vi "TimeFlow_for_泰克.vi"() -> ()   [LabVIEW 2017]
uses:
  <vilib>/vision/Image Controls.llb/IMAQ Image.ctl
  <vilib>/userdefined/High Color/IMAQdx.ctl
  <vilib>/vision/driver/IMAQdx.llb/IMAQdx Camera Control Mode.ctl
  <vilib>/Utility/file.llb/Write Delimited Spreadsheet (I64).vi
  <vilib>/vision/driver/NI_Vision_Acquisition_Software.lvlib
  <vilib>/vision/NI_Vision_Development_Module.lvlib
panel:
  in  "EOT reset":bool=TRUE
  out "DO 4":bool
  out "DO 2":bool
  out "DO 0":bool
  out "None":dbl
  out "Total":dbl
  out "No sample":dbl
  out "NG":dbl
  out "PASS":dbl
  in  "SOT single trigger":bool
  in  "SOT inverse":bool
  out "code":u32
  in  "Camera port":T1="cam1"
  in  "No sample":bool
  in  "NG":bool
  in  "EOT inverse":bool
  out "EOT":bool
  in  "CCD 啟動":bool
  out "EOT切換2":bool
  out "結果":bool
  out "檢查":bool
  out "EOT切換1":bool
  out "SOT等待":bool
  out "SOT":bool
  in  "EOT Run End":bool=TRUE
  in  "EOT Run State":bool
  in  "EOT Start State":bool=TRUE
  in  "physical channels":string="PCI-1730,BID#0"
  in  "儲存DATA":bool
  in  "儲存IMAGE":bool
  in  "清除":bool
  out "Show":u32[](graph)
  out "Time":T2
  in  "EOT DELAY":u32=20
  in  "Pass":bool=TRUE
  in  "虛擬檢測時間":u32=5
  in  "等待拍照":u32=13
  in  "SOT DELAY":u32
  in  "與機台連線":bool=TRUE
  out "New Image":T3
  in  "連續取像":bool=TRUE
  in  "Angle (degrees)":sgl format="%.2f"
  out "Image":T3(plugin-control)
  in  "error in":errorcluster
  in  "stop":bool
  out "IO status":bool
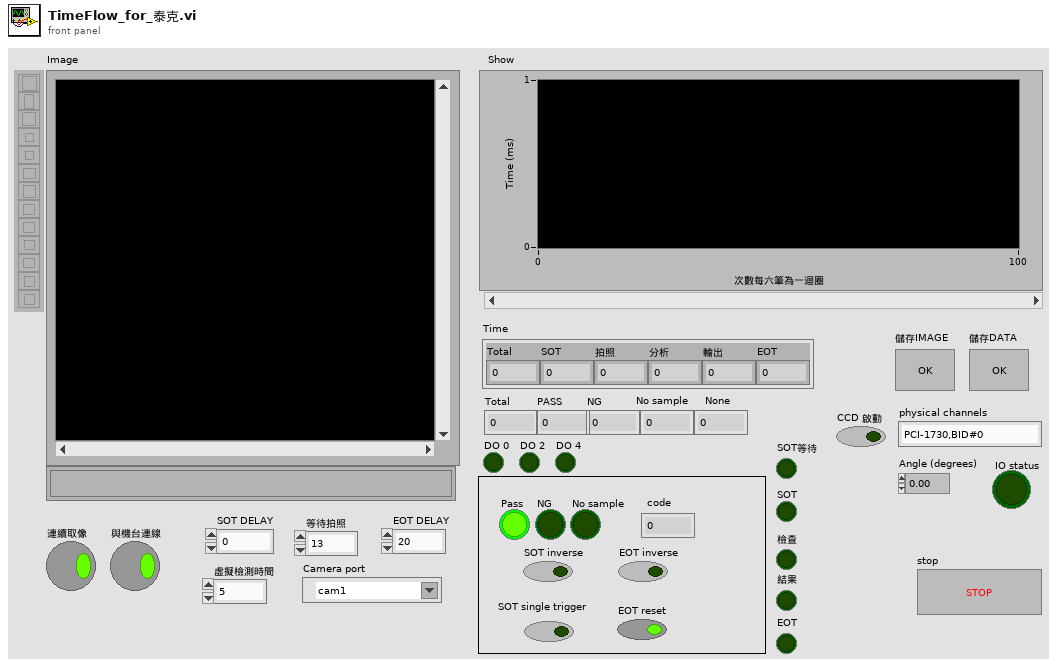
[diagram p1: front panel]
types:
  T1 = typedef "IMAQdx.ctl" = refnum<k21>
  T2 = cluster{"Total":dbl, "SOT":dbl, "拍照":dbl, "分析":dbl, "輸出":dbl, "EOT":dbl}
  T3 = typedef "IMAQ Image.ctl" = refnum<image>
  T4 = typedef "NI_Vision_Acquisition_Software.lvlib/IMAQdx Camera Control Mode.ctl" = enum32{"Controller", "Listener"}
  T5 = typedef "Image Type" = u32
  T6 = cluster{"task DI 0~7":i32, "portBit":i32, "Boolean out":bool}
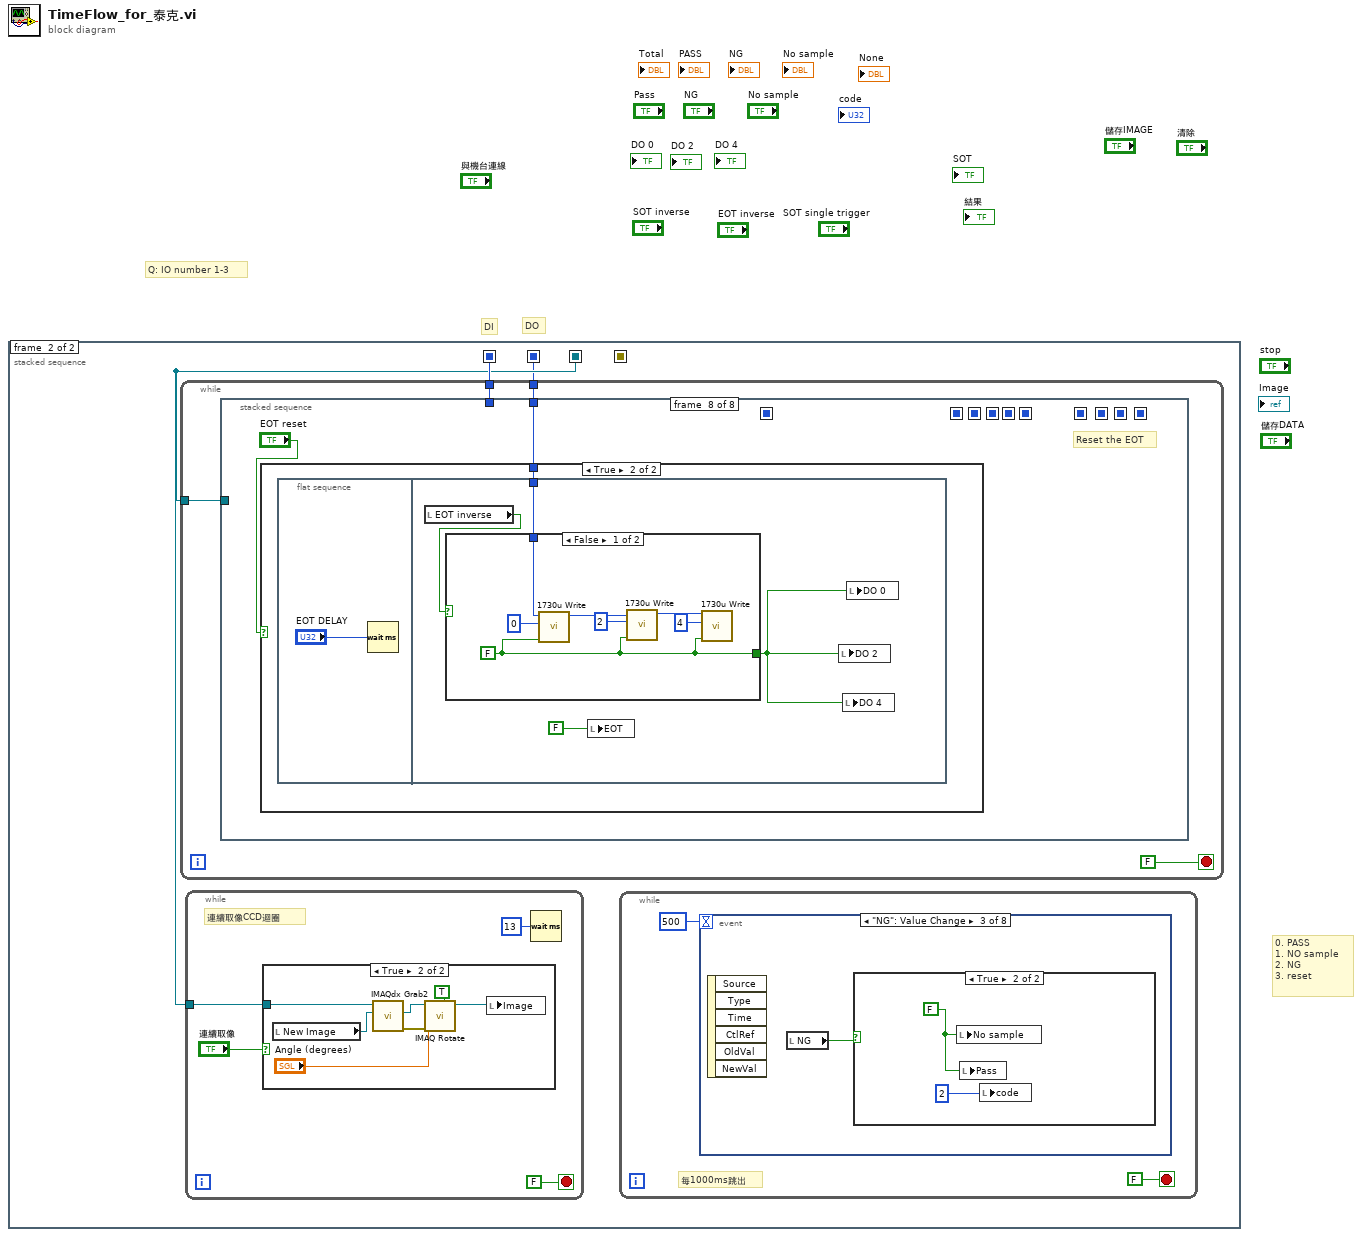
[diagram p0: block diagram]
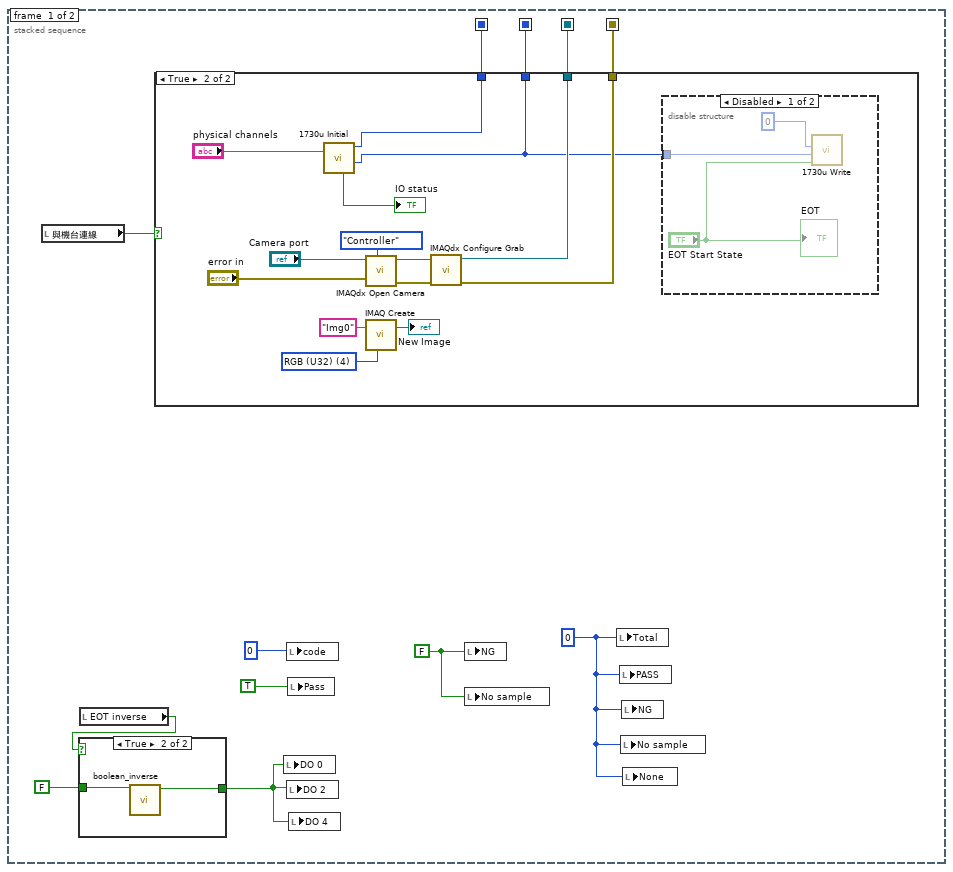
[diagram p2: hidden frame]
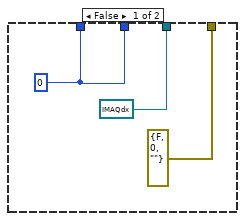
[diagram p4: hidden frame]
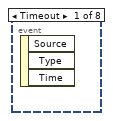
[diagram p6: hidden frame]
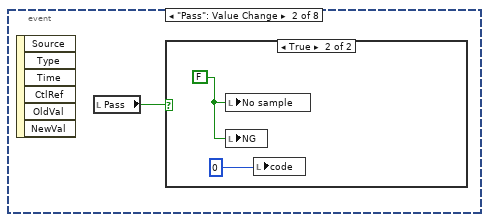
[diagram p7: hidden frame]
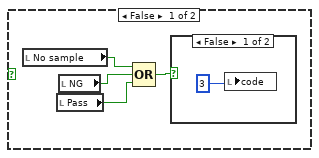
[diagram p8: hidden frame]
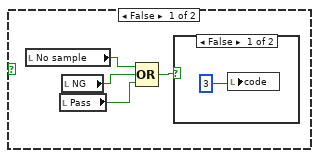
[diagram p10: hidden frame]
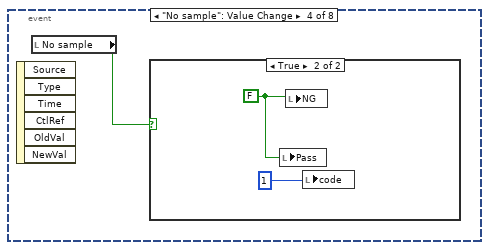
[diagram p12: hidden frame]
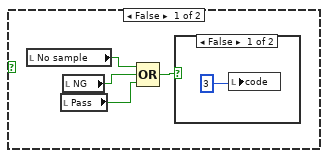
[diagram p13: hidden frame]
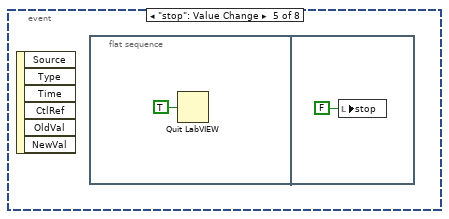
[diagram p15: hidden frame]
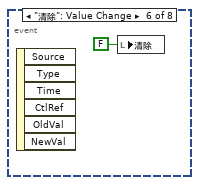
[diagram p16: hidden frame]
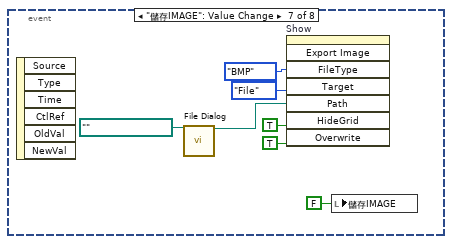
[diagram p17: hidden frame]
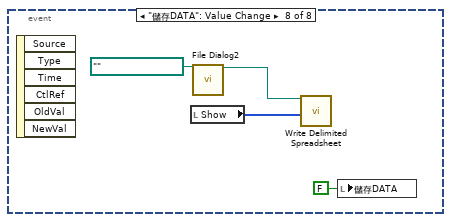
[diagram p18: hidden frame]
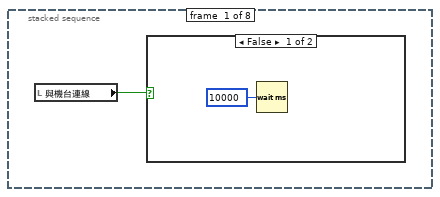
[diagram p20: hidden frame]
diagram:
  # "0. PASS\n1. NO sample\n2. NG\n3. reset"
  # "Q: IO number 1-3"
  # "DO"
  # "DI"
  n1 = stacked-sequence {
    seq-local: [w12 _] -> [_ w38]
    seq-local: [w9 _] -> [_ w36]
    seq-local: [w11 _] -> [_ _]
    seq-local: [w10 _] -> [_ w37]
    frame #0 {
      w5 = 0
      w8 = FALSE
      n2 = local read "與機台連線"() -> (w7:bool)
      n3 = local read "EOT inverse"() -> (w2:bool)
      n4 = case shown="True" w2 {
        tunnel: FALSE -> [w13 w15]
        tunnel: [w13 w14] -> w1
        frame False {
        }
        frame True {
          n5 = call "boolean_inverse.vi"("Boolean in"=w15) -> ("Boolean out"=w14:bool)  [unwired: 10 in]
        }
      }
      n6 = case shown="True" w7 {
        tunnel: [w18 w32] -> w12
        tunnel: [errorcluster {"status"=FALSE, "code"=0, "source"=""} ("error out") w31] -> w11
        tunnel: [T1 refnum ("Session Out") w30] -> w10
        tunnel: [w18 w29] -> w9
        frame False {
          w18 = 0
        }
        frame True {
          w21 = T5 4 items=["Grayscale (U8)", "Grayscale (I16)", "Grayscale (SGL)", "Complex (CSG)", "RGB (U32)", "HSL (U32)", "RGB (U64)", "Grayscale (U16)"] ("Image Type")
          n7 = call <userlib>:"1730u Initial.vi"("physical channels"="physical channels") -> ("task DO 0~7"=w29:i32, "task DI 0~7"=w32:i32, "status"=→"IO status":bool)  [unwired: 6 in, 2 out]
          n8 = call <vilib>:"IMAQdx Open Camera.vi"("Camera Control Mode"=IMAQdx_Camera_Control_Mode."Controller", "error in"="error in", "Session In"="Camera port") -> ("error out"=w25:errorcluster, "Session Out"=w26:T1)  [unwired: 7 in]
          n9 = call "IMAQ Create"("Image Name"="Img0", "Image Type"=w21) -> ("New Image"=→"New Image":T3)  [unwired: 3 in, 1 out]
          n10 = call <vilib>:"IMAQdx Configure Grab.vi"("error in"=w25, "Session In"=w26) -> ("error out"=w31:errorcluster, "Session Out"=w30:T1)  [unwired: 8 in]
          n11 = disable-structure shown="Disabled" {
            disable-tunnel: w29 -> [w34 _]
            frame Disabled {
              n12 = call <userlib>:"1730u Write.vi"("data"="EOT Start State", "portBit"=0, "DO task in"=w34) -> ()  [unwired: 8 in, 1 out]
              "EOT" <- "EOT Start State"
            }
            frame Enabled {
            }
          }
        }
      }
      n13 = local write "DO 0"(w1) -> ()
      n14 = local write "code"(0) -> ()
      n15 = local write "DO 2"(w1) -> ()
      n16 = local write "Pass"(TRUE) -> ()
      n17 = local write "DO 4"(w1) -> ()
      n18 = local write "NG"(w8) -> ()
      n19 = local write "No sample"(w8) -> ()
      n20 = local write "Total"(w5) -> ()
      n21 = local write "PASS"(w5) -> ()
      n22 = local write "No sample"(w5) -> ()
      n23 = local write "NG"(w5) -> ()
      n24 = local write "None"(w5) -> ()
    }
    frame #1 {
      n25 = while {
        tunnel: w38 -> [w92]
        tunnel: w37 -> [w91]
        tunnel: w36 -> [w90]
        stop <- FALSE stop-if-true
        n26 = stacked-sequence {
          seq-local: [_ w99 _ _ _ _ _ _] -> [_ _ w138 _ _ _ w269 _]
          seq-local: [_ _ w137 _ _ _ _ _] -> [_ _ _ _ _ _ w265 _]
          seq-local: [_ _ w136 _ _ _ _ _] -> [_ _ _ w145 _ _ _ _]
          seq-local: [_ _ _ w143 _ _ _ _] -> [_ _ _ _ _ _ w264 _]
          seq-local: [_ _ _ w141 _ _ _ _] -> [_ _ _ _ w189 _ _ _]
          seq-local: [_ _ _ _ w178 _ _ _] -> [_ _ _ _ _ w226 _ _]
          seq-local: [_ _ _ _ w188 _ _ _] -> [_ _ _ _ _ _ w263 _]
          seq-local: [_ _ _ _ w187 _ _ _] -> [_ _ _ _ _ w224 _ _]
          seq-local: [_ _ _ _ _ w223 _ _] -> [_ _ _ _ _ _ w262 _]
          seq-local: [_ _ _ _ _ w222 _ _] -> [_ _ _ _ _ _ w267 _]
          tunnel: w92 -> [_ w100 _ _ _ w219 _ _]
          tunnel: w91 -> [_ _ _ w148 _ _ _ _]
          tunnel: w90 -> [_ w98 _ _ w176 _ _ w271]
          frame #0 {
            n27 = local read "與機台連線"() -> (w94:bool)
            n28 = case shown="False" w94 {
              frame False {
                n29 = Wait (ms)(milliseconds to wait=u32 10000) -> ()  [unwired: 1 out]
              }
              frame True {
              }
            }
          }
          frame #1 {
            # "Double reset the EOT"
            # "IO"
            n30 = flat-sequence {
              tunnel: w100 -> [w103]
              tunnel: [w102] -> w99
              frame #0 {
                n31 = Wait (ms)(milliseconds to wait="SOT DELAY") -> ()  [unwired: 1 out]
              }
              frame #1 {
                n32 = while {
                  tunnel: w103 -> [w115]
                  tunnel: [w113] -> w102
                  stop <- w114 stop-if-true
                  n33 = call <userlib>:"1730u Read.vi"("portBit"=0, "DI task in"=w115) -> ("data"=w107:bool)  [unwired: 8 in, 1 out]
                  n34 = local write "EOT切換2"(FALSE ("EOT切換2")) -> ()
                  n35 = local read "SOT single trigger"() -> (w106:bool)
                  n36 = local read "SOT inverse"() -> (w108:bool)
                  n37 = case shown="True" w108 {
                    tunnel: w107 -> [w116 w118]
                    tunnel: [w116 w117] -> w105
                    frame False {
                    }
                    frame True {
                      n38 = call "boolean_inverse.vi"("Boolean in"=w118) -> ("Boolean out"=w117:bool)  [unwired: 10 in]
                    }
                  }
                  n39 = local read "與機台連線"() -> (w110:bool)
                  n40 = Or(x=w106, y=w105) -> (x .or. y?=w104:bool)
                  n41 = And(x=w104, y=w110) -> (x .and. y?=w114:bool)
                  n42 = local write "SOT"(w104) -> ()
                  n43 = case shown="True" w114 {
                    tunnel: [u32 0 ("millisecond timer value") w120] -> w113
                    frame False {
                    }
                    frame True {
                      n44 = Tick Count (ms)() -> (millisecond timer value=w120:u32)
                    }
                  }
                  "SOT等待" <- TRUE ("SOT等待")
                }
              }
            }
            n45 = local read "EOT inverse"() -> (w97:bool)
            n46 = case shown="False" w97 {
              tunnel: w98 -> [w122 w131]
              tunnel: [w121 w128] -> w96
              frame False {
                w121 = FALSE ("data")
                n47 = call <userlib>:"1730u Write.vi"("data"=w121, "portBit"=0, "DO task in"=w122) -> ("DO task out"=w127:i32)  [unwired: 8 in]
                n48 = call <userlib>:"1730u Write.vi"("data"=w121, "portBit"=2, "DO task in"=w127) -> ("DO task out"=w126:i32)  [unwired: 8 in]
                n49 = call <userlib>:"1730u Write.vi"("data"=w121, "portBit"=4, "DO task in"=w126) -> ()  [unwired: 8 in, 1 out]
              }
              frame True {
                w128 = TRUE ("data")
                n50 = call <userlib>:"1730u Write.vi"("data"=w128, "portBit"=0, "DO task in"=w131) -> ("DO task out"=w133:i32)  [unwired: 8 in]
                n51 = call <userlib>:"1730u Write.vi"("data"=w128, "portBit"=2, "DO task in"=w133) -> ("DO task out"=w129:i32)  [unwired: 8 in]
                n52 = call <userlib>:"1730u Write.vi"("data"=w128, "portBit"=4, "DO task in"=w129) -> ()  [unwired: 8 in, 1 out]
              }
            }
            n53 = local write "DO 2"(w96) -> ()
            n54 = local write "DO 0"(w96) -> ()
            n55 = local write "DO 4"(w96) -> ()
          }
          frame #2 {
            w135 = FALSE ("SOT等待")
            n56 = Wait (ms)(milliseconds to wait="等待拍照") -> ()  [unwired: 1 out]
            n57 = local write "SOT等待"(w135) -> ()
            n58 = local write "SOT single trigger"(w135) -> ()
            n59 = Tick Count (ms)() -> (millisecond timer value=w136:u32)
            n60 = Subtract(x=w136, y=w138) -> (x-y=w137:u32)
          }
          frame #3 {
            n61 = flat-sequence {
              tunnel: w148 -> [w156]
              tunnel: [w155] -> w147
              tunnel: [w154] -> w146
              tunnel: w145 -> [w153]
              tunnel: [w152] -> w144
              tunnel: [w151] -> w142
              tunnel: [w168] -> w143
              tunnel: [w166] -> w141
              tunnel: w142 -> [w166]
              tunnel: w144 -> [w168]
              tunnel: w146 -> [_]
              tunnel: w147 -> [w169]
              frame #0 {
                # "CCD"
                n62 = local read "New Image"() -> (w149:T3)
                n63 = case shown="True" "CCD 啟動" {
                  tunnel: w156 -> [_ w165]
                  tunnel: [w157 w161] -> w155
                  tunnel: [errorcluster {"status"=FALSE, "code"=0, "source"=""} ("error out") w160] -> w154
                  tunnel: w149 -> [w157 w159]
                  frame False {
                  }
                  frame True {
                    n64 = local read "Angle (degrees)"() -> (w162:sgl)
                    n65 = call <vilib>:"IMAQdx Grab2.vi"("Image In"=w159, "Session In"=w165) -> ("error out"=w163:errorcluster, "Image Out"=w164:T3)  [unwired: 6 in, 2 out]
                    n66 = call "IMAQ Rotate"("error in (no error)"=w163, "Angle (degrees)"=w162, "Image Src"=w164) -> ("error out"=w160:errorcluster, "Image Dst Out"=w161:T3)  [unwired: 7 in]
                  }
                }
                n67 = Tick Count (ms)() -> (millisecond timer value=w151:u32)
                n68 = Subtract(x=w151, y=w153) -> (x-y=w152:u32)
              }
              frame #1 {
                # "Set the runtime for algorithm"
                n69 = local write "Image"(w169) -> ()
                n70 = Wait (ms)(milliseconds to wait="虛擬檢測時間") -> ()  [unwired: 1 out]
              }
            }
            "檢查" <- TRUE ("檢查")
          }
          frame #4 {
            n71 = local read "code"() -> (w185:u32)
            n72 = local write "檢查"(FALSE ("檢查")) -> ()
            n73 = local write "結果"(TRUE ("結果")) -> ()
            n74 = case shown="0, Default" w185 {
              tunnel: [TRUE TRUE TRUE FALSE] -> w184
              tunnel: [FALSE TRUE TRUE FALSE] -> w183
              tunnel: [FALSE TRUE FALSE FALSE] -> w182
              frame 0, Default {
                n75 = local read "PASS"() -> (w200:dbl)
                n76 = Increment(x=w200) -> (x+1=w199:dbl)
                n77 = local write "PASS"(w199) -> ()
              }
              frame 1 {
                n78 = local read "No sample"() -> (w204:dbl)
                n79 = Increment(x=w204) -> (x+1=w205:dbl)
                n80 = local write "No sample"(w205) -> ()
              }
              frame 2 {
                n81 = local read "NG"() -> (w210:dbl)
                n82 = Increment(x=w210) -> (x+1=w209:dbl)
                n83 = local write "NG"(w209) -> ()
              }
              frame 3 {
                n84 = local read "None"() -> (w214:dbl)
                n85 = Increment(x=w214) -> (x+1=w215:dbl)
                n86 = local write "None"(w215) -> ()
              }
            }
            n87 = local read "EOT inverse"() -> (w177:bool)
            n88 = case shown="True" w177 {
              tunnel: w184 -> [w192 w198]
              tunnel: [w192 w197] -> w170
              tunnel: w183 -> [w191 w196]
              tunnel: [w191 w195] -> w171
              tunnel: w182 -> [w190 w194]
              tunnel: [w190 w193] -> w172
              frame False {
              }
              frame True {
                n89 = call "boolean_inverse.vi"("Boolean in"=w198) -> ("Boolean out"=w197:bool)  [unwired: 10 in]
                n90 = call "boolean_inverse.vi"("Boolean in"=w196) -> ("Boolean out"=w195:bool)  [unwired: 10 in]
                n91 = call "boolean_inverse.vi"("Boolean in"=w194) -> ("Boolean out"=w193:bool)  [unwired: 10 in]
              }
            }
            n92 = call <userlib>:"1730u Write.vi"("data"=w172, "portBit"=4, "DO task in"=w176) -> ()  [unwired: 8 in, 1 out]
            n93 = call <userlib>:"1730u Write.vi"("data"=w171, "portBit"=2, "DO task in"=w176) -> ()  [unwired: 8 in, 1 out]
            n94 = call <userlib>:"1730u Write.vi"("data"=w170, "portBit"=0, "DO task in"=w176) -> ("DO task out"=w178:i32)  [unwired: 8 in]
            n95 = local write "DO 2"(w171) -> ()
            n96 = local write "DO 4"(w172) -> ()
            n97 = local write "DO 0"(w170) -> ()
            n98 = Tick Count (ms)() -> (millisecond timer value=w187:u32)
            n99 = Subtract(x=w187, y=w189) -> (x-y=w188:u32)
            n100 = local read "Total"() -> (w173:dbl)
            n101 = Increment(x=w173) -> (x+1=w174:dbl)
            n102 = local write "Total"(w174) -> ()
          }
          frame #5 {
            n103 = flat-sequence {
              tunnel: w219 -> [w229]
              tunnel: w226 -> [w228]
              tunnel: [w227] -> w221
              tunnel: [w229] -> w220
              tunnel: [w235] -> w225
              tunnel: w221 -> [w236]
              tunnel: w220 -> [w235]
              tunnel: w225 -> [w248]
              frame #0 {
                n104 = disable-structure shown="Disabled" {
                  disable-tunnel: w228 -> [w232 _]
                  disable-tunnel: [w231 _] -> w227
                  frame Disabled {
                    n105 = local write "EOT"("EOT Run State") -> ()
                    n106 = call <userlib>:"1730u Write.vi"("data"="EOT Run State", "portBit"=0, "DO task in"=w232) -> ("DO task out"=w231:i32)  [unwired: 8 in]
                    "EOT切換1" <- TRUE ("EOT切換1")
                  }
                  frame Enabled {
                  }
                }
              }
              frame #1 {
                n107 = disable-structure shown="Disabled" {
                  disable-tunnel: w236 -> [w240 _]
                  frame Disabled {
                    n108 = local write "結果"(FALSE ("結果")) -> ()
                    n109 = local write "EOT"("EOT Run End") -> ()
                    n110 = call <userlib>:"1730u Write.vi"("data"="EOT Run End", "portBit"=0, "DO task in"=w240) -> ()  [unwired: 8 in, 1 out]
                    "EOT切換2" <- TRUE ("EOT切換2")
                  }
                  frame Enabled {
                  }
                }
              }
              frame #2 {
                n111 = local read "SOT inverse"() -> (w244:bool)
                n112 = case shown="True" w244 {
                  tunnel: FALSE -> [w254 w256]
                  tunnel: [w254 w255] -> w243
                  frame False {
                  }
                  frame True {
                    n113 = call "boolean_inverse.vi"("Boolean in"=w256) -> ("Boolean out"=w255:bool)  [unwired: 10 in]
                  }
                }
                n114 = Bundle("task DI 0~7"=w248, "portBit"=0, "Boolean out"=w243) -> (w247:T6)  [unwired: 1 in]
                n115 = local write "EOT"(TRUE ("EOT切換1")) -> ()
                n116 = call <userlib>:"Check DI State 1730u.vi"("Time Out"=u32 3000 ("DI Time Out"), "Scan time"=u32 2 ("DI Scan time"), "Mode"=enum16{"Check One DI", "Check Two DI"}."Check One DI", "1 DI Mode"=w247) -> ("Finish?"=w253:bool)  [unwired: 7 in]
                n117 = local write "結果"(FALSE) -> ()
                n118 = case shown="True" w253 {
                  frame False {
                    n119 = One Button Dialog(message="SOT持續超過3秒\n沒有關閉") -> ()  [unwired: 1 in, 1 out]
                  }
                  frame True {
                    n120 = local write "SOT"(FALSE ("檢查")) -> ()
                  }
                }
              }
            }
            n121 = Tick Count (ms)() -> (millisecond timer value=w222:u32)
            n122 = Subtract(x=w222, y=w224) -> (x-y=w223:u32)
          }
          frame #6 {
            n123 = Tick Count (ms)() -> (millisecond timer value=w268:u32)
            n124 = Subtract(x=w268, y=w269) -> (x-y=w266:u32)
            n125 = Subtract(x=w268, y=w267) -> (x-y=w261:u32)
            n126 = Bundle(w266, w265, w264, w263, w262, w261) -> (w260:cluster{u32, u32, u32, u32, u32, u32})  [unwired: 1 in]
            "Time" <- w260
            n127 = Cluster To Array(cluster=w260) -> (array=→"Show":u32[])
          }
          frame #7 {
            # "Reset the EOT"
            n128 = case shown="True" "EOT reset" {
              tunnel: w271 -> [_ w272]
              frame False {
              }
              frame True {
                n129 = flat-sequence {
                  tunnel: w272 -> [w277]
                  frame #0 {
                    n130 = Wait (ms)(milliseconds to wait="EOT DELAY") -> ()  [unwired: 1 out]
                  }
                  frame #1 {
                    n131 = local read "EOT inverse"() -> (w276:bool)
                    n132 = case shown="False" w276 {
                      tunnel: w277 -> [w279 w286]
                      tunnel: [w278 w285] -> w274
                      frame False {
                        w278 = FALSE ("data")
                        n133 = call <userlib>:"1730u Write.vi"("data"=w278, "portBit"=0, "DO task in"=w279) -> ("DO task out"=w284:i32)  [unwired: 8 in]
                        n134 = call <userlib>:"1730u Write.vi"("data"=w278, "portBit"=2, "DO task in"=w284) -> ("DO task out"=w283:i32)  [unwired: 8 in]
                        n135 = call <userlib>:"1730u Write.vi"("data"=w278, "portBit"=4, "DO task in"=w283) -> ()  [unwired: 8 in, 1 out]
                      }
                      frame True {
                        w285 = TRUE ("data")
                        n136 = call <userlib>:"1730u Write.vi"("data"=w285, "portBit"=0, "DO task in"=w286) -> ("DO task out"=w291:i32)  [unwired: 8 in]
                        n137 = call <userlib>:"1730u Write.vi"("data"=w285, "portBit"=2, "DO task in"=w291) -> ("DO task out"=w290:i32)  [unwired: 8 in]
                        n138 = call <userlib>:"1730u Write.vi"("data"=w285, "portBit"=4, "DO task in"=w290) -> ()  [unwired: 8 in, 1 out]
                      }
                    }
                    n139 = local write "EOT"(FALSE ("EOT切換1")) -> ()
                    n140 = local write "DO 2"(w274) -> ()
                    n141 = local write "DO 4"(w274) -> ()
                    n142 = local write "DO 0"(w274) -> ()
                  }
                }
              }
            }
          }
        }
      }
      n143 = while {
        tunnel: w37 -> [w79]
        stop <- FALSE stop-if-true
        # "連續取像CCD迴圈"
        n144 = case shown="True" "連續取像" {
          tunnel: w79 -> [_ w85]
          frame False {
          }
          frame True {
            n145 = local read "New Image"() -> (w84:T3)
            n146 = call <vilib>:"IMAQdx Grab2.vi"("Image In"=w84, "Session In"=w85) -> ("error out"=w89:errorcluster, "Image Out"=w88:T3)  [unwired: 6 in, 2 out]
            n147 = call "IMAQ Rotate"("Maintain Size"=TRUE, "error in (no error)"=w89, "Angle (degrees)"="Angle (degrees)", "Image Src"=w88) -> ("Image Dst Out"=w86:T3)  [unwired: 6 in, 1 out]
            n148 = local write "Image"(w86) -> ()
          }
        }
        n149 = Wait (ms)(milliseconds to wait=u32 13) -> ()  [unwired: 1 out]
      }
      n150 = while {
        stop <- FALSE stop-if-true
        # "每1000ms跳出"
        n151 = event shown="[2] \"NG\": Value Change" {
          selector: _ -> [_ _ _ _ _ _ _ _]
          dyn-events: _ -> [_ _ _ _ _ _ _ _]
          timeout: 500 -> [_ _ _ _ _ _ _ _]
          event Timeout {
            n152 = event-data() -> ()  [unwired: 1 in, 3 out]
          }
          event "Pass": Value Change {
            n153 = event-data() -> ()  [unwired: 1 in, 6 out]
            n154 = local read "Pass"() -> (w41:bool)
            n155 = case shown="True" w41 {
              frame False {
                n156 = local read "No sample"() -> (w43:bool)
                n157 = local read "Pass"() -> (w45:bool)
                n158 = local read "NG"() -> (w44:bool)
                n159 = Compound Arithmetic op=OR(w43, w44, w45) -> (w42:bool)
                n160 = case shown="False" w42 {
                  frame False {
                    n161 = local write "code"(3) -> ()
                  }
                  frame True {
                  }
                }
              }
              frame True {
                w48 = FALSE
                n162 = local write "No sample"(w48) -> ()
                n163 = local write "NG"(w48) -> ()
                n164 = local write "code"(0) -> ()
              }
            }
          }
          event "NG": Value Change {
            n165 = event-data() -> ()  [unwired: 1 in, 6 out]
            n166 = local read "NG"() -> (w49:bool)
            n167 = case shown="True" w49 {
              frame False {
                n168 = local read "No sample"() -> (w51:bool)
                n169 = local read "Pass"() -> (w53:bool)
                n170 = local read "NG"() -> (w52:bool)
                n171 = Compound Arithmetic op=OR(w51, w52, w53) -> (w50:bool)
                n172 = case shown="False" w50 {
                  frame False {
                    n173 = local write "code"(3) -> ()
                  }
                  frame True {
                  }
                }
              }
              frame True {
                w56 = FALSE
                n174 = local write "No sample"(w56) -> ()
                n175 = local write "Pass"(w56) -> ()
                n176 = local write "code"(2) -> ()
              }
            }
          }
          event "No sample": Value Change {
            n177 = event-data() -> ()  [unwired: 1 in, 6 out]
            n178 = local read "No sample"() -> (w57:bool)
            n179 = case shown="True" w57 {
              frame False {
                n180 = local read "No sample"() -> (w59:bool)
                n181 = local read "Pass"() -> (w61:bool)
                n182 = local read "NG"() -> (w60:bool)
                n183 = Compound Arithmetic op=OR(w59, w60, w61) -> (w58:bool)
                n184 = case shown="False" w58 {
                  frame False {
                    n185 = local write "code"(3) -> ()
                  }
                  frame True {
                  }
                }
              }
              frame True {
                w64 = FALSE
                n186 = local write "Pass"(w64) -> ()
                n187 = local write "NG"(w64) -> ()
                n188 = local write "code"(1) -> ()
              }
            }
          }
          event "stop": Value Change {
            n189 = event-data() -> ()  [unwired: 1 in, 6 out]
            n190 = flat-sequence {
              frame #0 {
                n191 = Quit LabVIEW(quit? (T)=TRUE) -> ()
              }
              frame #1 {
                n192 = local write "stop"(FALSE ("stop")) -> ()
              }
            }
          }
          event "清除": Value Change {
            n193 = event-data() -> ()  [unwired: 1 in, 6 out]
            n194 = local write "清除"(FALSE ("清除")) -> ()
          }
          event "儲存IMAGE": Value Change {
            n195 = event-data() -> ()  [unwired: 1 in, 6 out]
            n196 = call "File Dialog"("start path"=path "") -> ("selected path"=w69:path)  [unwired: 11 in, 3 out]
            n197 = invoke on="Show" class="WFChart (strict)" method="Export Image"("FileType"=enum32{"BMP", "EPS", "EMF", "PICT"}."BMP" ("File Type"), "Target"=enum32{"File", "Clipboard"}."File", "Path"=w69, "HideGrid"=TRUE ("Hide Grid"), "Overwrite"=TRUE ("Always Overwrite")) -> ()  [unwired: 3 in, 8 out]
            n198 = local write "儲存IMAGE"(FALSE ("儲存")) -> ()
          }
          event "儲存DATA": Value Change {
            n199 = event-data() -> ()  [unwired: 1 in, 6 out]
            n200 = local read "Show"() -> (w77:u32[])
            n201 = call "File Dialog2"("start path"=path "") -> ("selected path"=w76:path)  [unwired: 11 in, 3 out]
            n202 = call-poly <vilib>:"Write Delimited Spreadsheet.vi"("file path (dialog if empty)"=w76, "1D data"=w77) -> ()  [unwired: 12 in, 2 out]
            n203 = local write "儲存DATA"(FALSE ("儲存DATA")) -> ()
          }
        }
      }
    }
  }
